vi "PID_controller.vi"(4 "Kd/Tau":fxp<+/-,32,6>, 5 "Ki*Tau":fxp<+/-,32,6>, 6 "Kp":fxp<+/-,32,6>, 7 "Reset":bool=TRUE, 8 "input valid":bool=TRUE, 9 "Enabled":bool=TRUE, 10 "Y in":fxp<+/-,32,14>, 11 "Ref in":fxp<+/-,32,14>) -> (0 "output valid":bool, 2 "Y out":fxp<+/-,32,14>, 3 "e(n)":fxp<+/-,32,14>)   [LabVIEW 2018]
uses:
  <vilib>/rvi/FXPMathLib/FxpConvert/subVIs/nifxpmath_Convert_SimConfig.ctl
  <vilib>/fxp/LVFixedPointQuantizationPolicyTypeDef.ctl
  <vilib>/fxp/LVFixedPointOverflowPolicyTypeDef.ctl
  <vilib>/rvi/FXPMathLib/FxpConvert/simVIs/DllFxpConvertTemp_sub.vi
  <vilib>/rvi/FXPMathLib/FxpSub/XNode/nifxpmath_Sub.xnode
  <vilib>/rvi/FXPMathLib/FxpAdd/XNode/nifxpmath_Add.xnode
  <vilib>/rvi/FXPMathLib/FxpConvert/XNode/nifxpmath_Convert.xnode
  <vilib>/rvi/FXPMathLib/FxpMul/XNode/nifxpmath_Multiplier.xnode
  <vilib>/rvi/FXPMathLib/sim/FxpSim.dll
panel:
  out "Ref out":fxp<+/-,32,14>
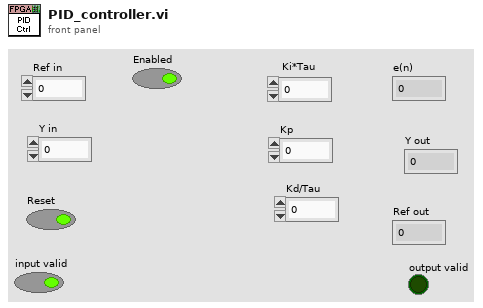
[diagram p1: front panel]
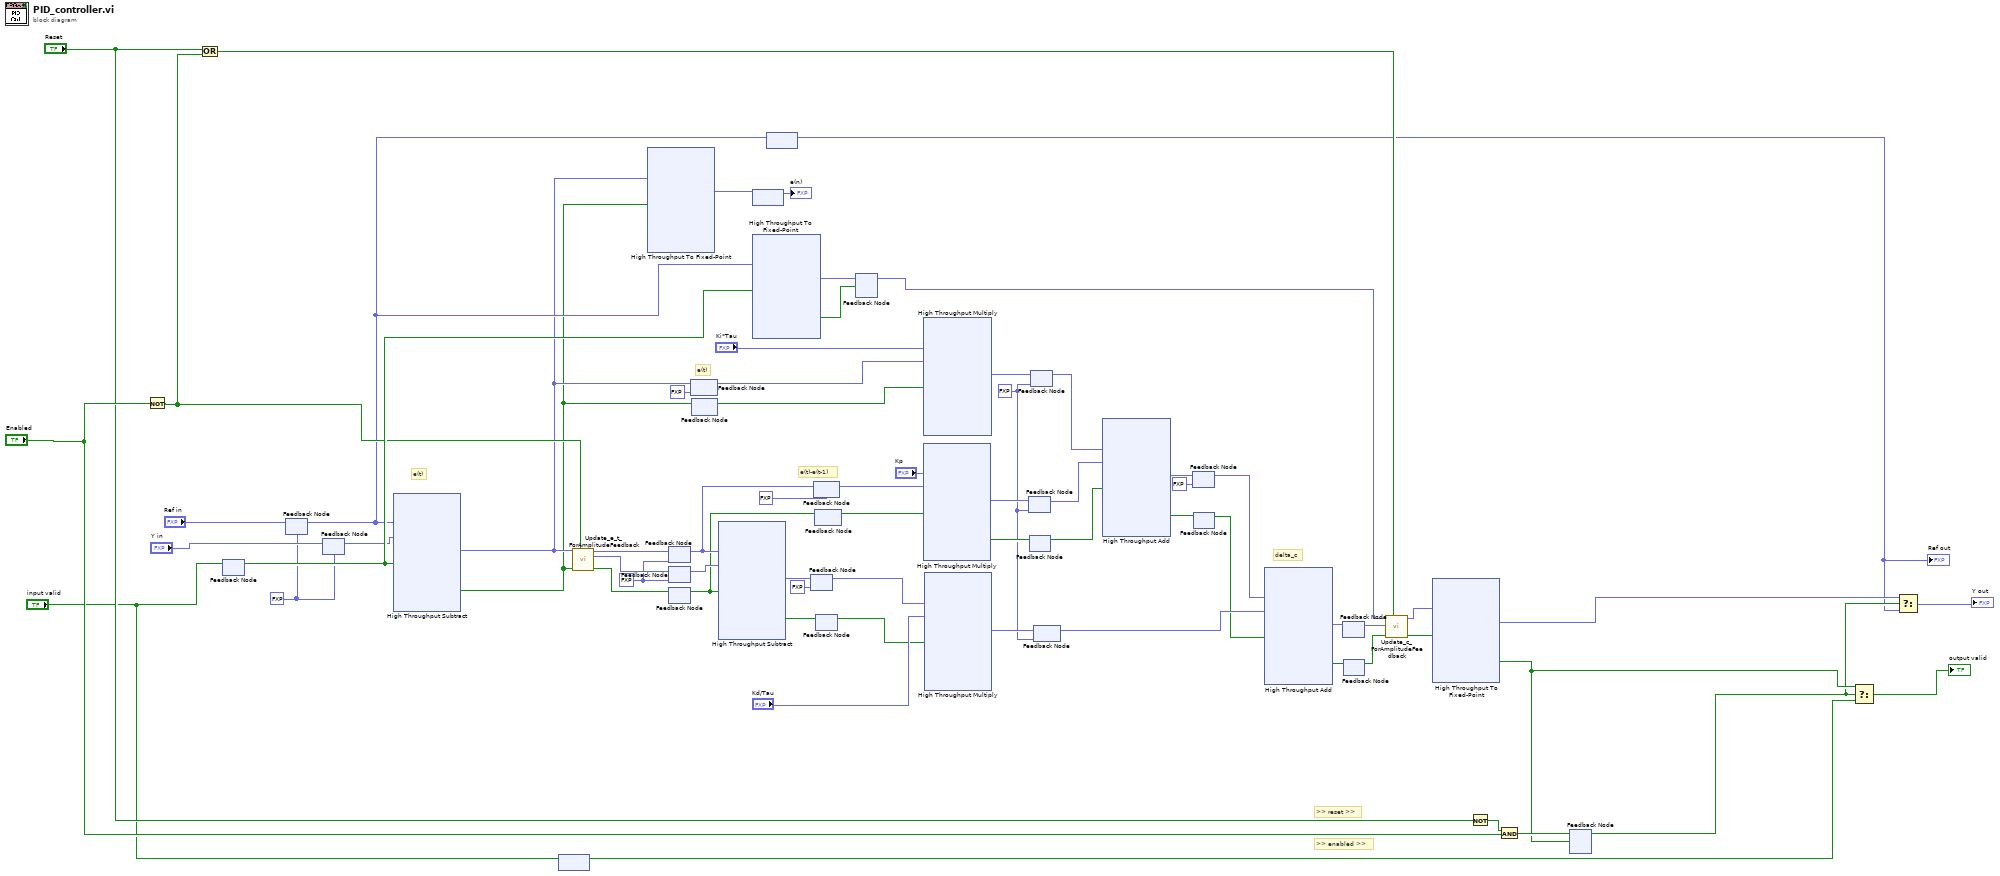
[diagram p0: block diagram]
diagram:
  w7 = fxp<+/-,34,16> 0.0 ("e(t-1)-e(t-2)")
  w27 = fxp<+/-,32,14> 0.0 ("Ref in")
  w48 = fxp<+/-,32,21> 0.0 ("x*y")
  # ">> reset >>"
  # ">> enabled >>"
  # "delta_c"
  # "e(t)-e(t-1)"
  # "e(t)"
  # "e(t)"
  n1 = Not(x="Enabled") -> (.not. x?=w33:bool)
  n2 = Or(x="Reset", y=w33) -> (x .or. y?=w32:bool)
  n3 = feedback #1() -> (w34:bool)  [unwired: 1 in]
  n4 = feedback-in #1("input valid") -> ()
  n5 = feedback-in #2("Ref in") -> ()
  n6 = feedback #2(w27) -> (w13:fxp<+/-,32,14>)
  n7 = feedback #3(w27) -> (w28:fxp<+/-,32,14>)
  n8 = feedback-in #3("Y in") -> ()
  n9 = xnode "High Throughput Subtract"("x"=w13, "y"=w28, "input valid"=w34) -> ("x-y"=w2:fxp<+/-,33,15>, "output valid"=w1:bool)  [unwired: 1 in, 1 out]
  n10 = feedback #4() -> (w8:bool)  [unwired: 1 in]
  n11 = feedback-in #4("input valid") -> ()
  n12 = call "Update_e_t_ForAmplitudeFeedback.vi"("Rest"=w33, "input valid"=w1, "e(t)"=w2) -> ("output valid"=w35:bool, "e(t-1)-e(t-2)"=w42:fxp<+/-,34,16>, "e(t)-e(t-1)"=w39:fxp<+/-,34,16>)  [unwired: 6 in]
  n13 = xnode "High Throughput To Fixed-Point"("x"=w2, "input valid"=w1) -> ("y"=w4:fxp<+/-,32,14>)  [unwired: 1 in, 2 out]
  n14 = feedback #5(w7) -> (w49:fxp<+/-,34,16>)
  n15 = feedback-in #5(w39) -> ()
  n16 = feedback #6(w7) -> (w68:fxp<+/-,34,16>)
  n17 = feedback-in #6(w42) -> ()
  n18 = feedback #7() -> (w36:bool)  [unwired: 1 in]
  n19 = feedback-in #7(w35) -> ()
  n20 = feedback #8(fxp<+/-,33,15> 0.0 ("x-y")) -> (w62:fxp<+/-,33,15>)
  n21 = feedback-in #8(w2) -> ()
  n22 = feedback #9() -> (w60:bool)  [unwired: 1 in]
  n23 = feedback-in #9(w1) -> ()
  n24 = xnode "High Throughput Subtract"("x"=w49, "y"=w68, "input valid"=w36) -> ("x-y"=w66:fxp<+/-,35,17>, "output valid"=w65:bool)  [unwired: 1 in, 1 out]
  n25 = feedback #10() -> (→"e(n)":fxp<+/-,32,14>)  [unwired: 1 in]
  n26 = feedback-in #10(w4) -> ()
  n27 = xnode "High Throughput To Fixed-Point"("x"=w13, "input valid"=w34) -> ("y"=w19:fxp<+/-,32,21>, "output valid"=w20:bool)  [unwired: 1 in, 1 out]
  n28 = feedback #11() -> (w10:fxp<+/-,32,14>)  [unwired: 1 in]
  "Ref out" <- w10
  n29 = feedback-in #11(w13) -> ()
  n30 = feedback #12(fxp<+/-,35,17> 0.0 ("x-y")) -> (w64:fxp<+/-,35,17>)
  n31 = feedback-in #12(w66) -> ()
  n32 = feedback #13(fxp<+/-,34,16> 0.0 ("e(t-1)-e(t-2)")) -> (w41:fxp<+/-,34,16>)
  n33 = feedback-in #13(w49) -> ()
  n34 = feedback #14() -> (w40:bool)  [unwired: 1 in]
  n35 = feedback-in #14(w36) -> ()
  n36 = feedback #15() -> (w61:bool)  [unwired: 1 in]
  n37 = feedback-in #15(w65) -> ()
  n38 = feedback #16() -> (w14:fxp<+/-,32,21>)  [unwired: 1 in]
  n39 = feedback-in #16(w19, w20) -> ()
  n40 = xnode ("High Throughput Multiply")("x"="Kp", "y"=w41, "input valid"=w40) -> ("x*y"=w57:fxp<+/-,32,21>, "output valid"=w56:bool)  [unwired: 1 in, 1 out]
  n41 = xnode ("High Throughput Multiply")("x"="Ki*Tau", "y"=w62, "input valid"=w60) -> ("x*y"=w59:fxp<+/-,32,21>)  [unwired: 1 in, 2 out]
  n42 = xnode ("High Throughput Multiply")("x"=w64, "y"="Kd/Tau", "input valid"=w61) -> ("x*y"=w55:fxp<+/-,32,21>)  [unwired: 1 in, 2 out]
  n43 = feedback #17(w48) -> (w24:fxp<+/-,32,21>)
  n44 = feedback-in #17(w57) -> ()
  n45 = feedback #18() -> (w23:bool)  [unwired: 1 in]
  n46 = feedback-in #18(w56) -> ()
  n47 = feedback #19(w48) -> (w58:fxp<+/-,32,21>)
  n48 = feedback-in #19(w59) -> ()
  n49 = feedback #20(w48) -> (w54:fxp<+/-,32,21>)
  n50 = feedback-in #20(w55) -> ()
  n51 = xnode ("High Throughput Add")("x"=w58, "y"=w24, "input valid"=w23) -> ("x+y"=w53:fxp<+/-,32,21>, "output valid"=w52:bool)  [unwired: 1 in, 1 out]
  n52 = feedback #21(fxp<+/-,32,21> 0.0 ("x+y")) -> (w51:fxp<+/-,32,21>)
  n53 = feedback-in #21(w53) -> ()
  n54 = feedback #22() -> (w50:bool)  [unwired: 1 in]
  n55 = feedback-in #22(w52) -> ()
  n56 = xnode ("High Throughput Add")("x"=w51, "y"=w54, "input valid"=w50) -> ("x+y"=w44:fxp<+/-,32,21>, "output valid"=w43:bool)  [unwired: 1 in, 1 out]
  n57 = feedback #23() -> (w26:fxp<+/-,32,21>)  [unwired: 1 in]
  n58 = feedback-in #23(w44) -> ()
  n59 = feedback #24() -> (w25:bool)  [unwired: 1 in]
  n60 = feedback-in #24(w43) -> ()
  n61 = call "Update_c_ForAmplitudeFeedback.vi"("Reset"=w32, "input valid"=w25, "delta_c"=w26, "reset value"=w14) -> ("output valid"=w17:bool, "c out"=w18:fxp<+/-,32,21>)  [unwired: 6 in]
  n62 = xnode "High Throughput To Fixed-Point"("x"=w18, "input valid"=w17) -> ("y"=w15:fxp<+/-,32,14>, "output valid"=w16:bool)  [unwired: 1 in, 1 out]
  n63 = Not(x="Reset") -> (.not. x?=w37:bool)
  n64 = And(x=w37, y="Enabled") -> (x .and. y?=w31:bool)
  n65 = feedback #25() -> (w12:bool)  [unwired: 1 in]
  n66 = feedback-in #25(w31, w16) -> ()
  n67 = Select(t=w16, s=w12, f=w8) -> (s? t:f=→"output valid":bool)
  n68 = Select(t=w15, s=w12, f=w10) -> (s? t:f=→"Y out":fxp<+/-,32,14>)
